vi "Convert Data Bytes to Motor Position.vi"(8 "DATA[7]":u8 format="%.0x", 9 "DATA[6]":u8 format="%.0x", 10 "DATA[5]":u8 format="%.0x", 11 "DATA[4]":u8 format="%.0x") -> (3 "Motor Position":sgl[](array[numeric]))   [LabVIEW 2025]
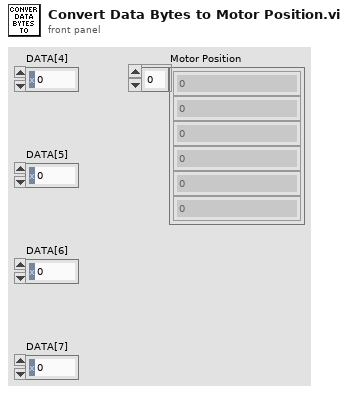
[diagram p1: front panel]
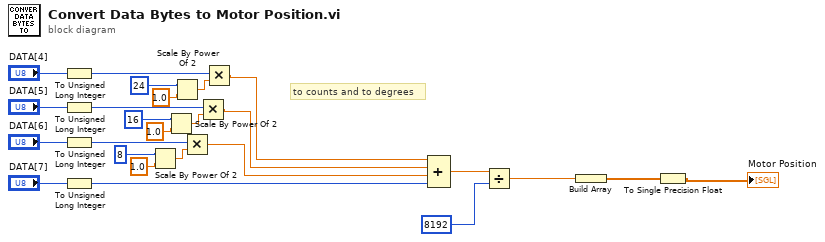
[diagram p0: block diagram]
diagram:
  # "to counts and to degrees"
  n1 = To Unsigned Long Integer(number="DATA[4]") -> (unsigned 32bit integer=w2:u32)
  n2 = To Unsigned Long Integer(number="DATA[5]") -> (unsigned 32bit integer=w7:u32)
  n3 = To Unsigned Long Integer(number="DATA[6]") -> (unsigned 32bit integer=w15:u32)
  n4 = To Unsigned Long Integer(number="DATA[7]") -> (unsigned 32bit integer=w16:u32)
  n5 = Scale By Power Of 2(n=i16 8, x=1.0) -> (x*2^n=w11:dbl)
  n6 = Scale By Power Of 2(n=i16 16, x=1.0) -> (x*2^n=w10:dbl)
  n7 = Scale By Power Of 2(n=i16 24, x=1.0) -> (x*2^n=w3:dbl)
  n8 = Multiply(x=w15, y=w11) -> (x*y=w14:dbl)
  n9 = Multiply(x=w7, y=w10) -> (x*y=w6:dbl)
  n10 = Multiply(x=w2, y=w3) -> (x*y=w1:dbl)
  n11 = Compound Arithmetic op=ADD(w1, w6, w14, w16) -> (w21:dbl)
  n12 = Divide(x=w21, y=u16 8192) -> (x/y=w19:dbl)
  n13 = Build Array(w19) -> (w18:dbl[])
  n14 = To Single Precision Float(number=w18) -> (single precision float=→"Motor Position":sgl[])
